vi "Picolog Channel Name.vi"(8 "Error In":errorcluster, 9 "Temperature Waveforms":waveform(dbl)[](array[waveform]), 10 "Channels":i16[](array[numeric])) -> (0 "Error Out":errorcluster, 1 "Temperature Waveforms with Names":waveform(dbl)[](array[waveform]))   [LabVIEW 2017]
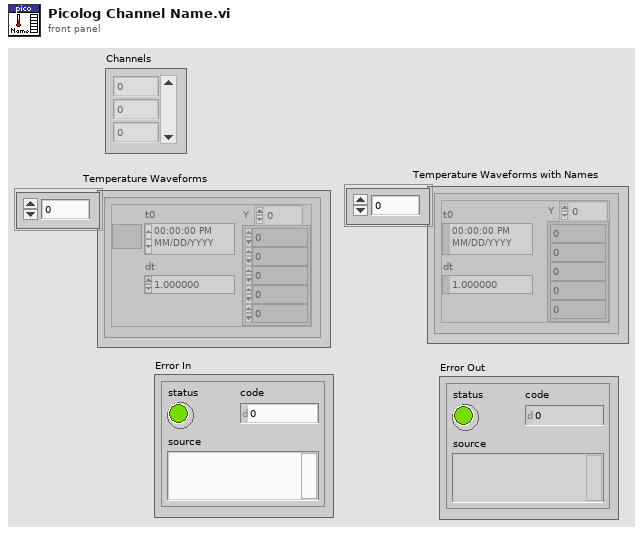
[diagram p1: front panel]
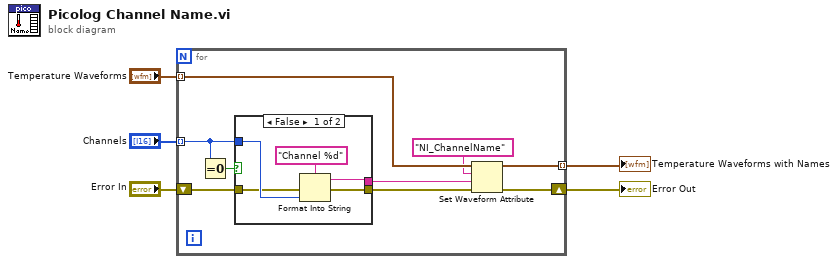
[diagram p0: block diagram]
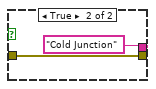
[diagram p2: hidden frame]
diagram:
  n1 = for {
    tunnel: "Temperature Waveforms" -> [w9] mode=indexing
    tunnel: [w8] -> w2 mode=indexing
    tunnel: "Channels" -> [w7] mode=indexing
    shift-right: [w14] -> w5
    shift-left: "Error In" -> [w12]
    n2 = Equal To 0?(x=w7) -> (x = 0?=w13:bool)
    n3 = case shown="False" w13 {
      tunnel: w7 -> [w18 _]
      tunnel: [w17 w20] -> w11
      tunnel: w12 -> [w16 w20]
      tunnel: [w15 "Cold Junction" ("format string")] -> w10
      frame False {
        n4 = Format Into String(format string="Channel %d", error in=w16, w18) -> (resulting string=w15:string, error out=w17:errorcluster)  [unwired: 1 in]
      }
      frame True {
      }
    }
    n5 = Set Waveform Attribute(4:w11, 5:w10, 6:"NI_ChannelName" ("name"), 7:w9) -> (0:w14:errorcluster, 3:w8:waveform(dbl))  [unwired: 1 out]
  }
  "Error Out" <- w5
  "Temperature Waveforms with Names" <- w2
